vi "Perform Action.vi"(8 "error in (no error)":errorcluster, 10 "Input":variant, 11 "DIO DAQmx Fixed Freq PWM CFG in":refnum<class "CO DAQmx Fixed Freq PWM CFG.lvclass">) -> (0 "error out":errorcluster, 2 "Output":variant, 3 "DIO DAQmx Fixed Freq PWM CFG out":refnum<class "CO DAQmx Fixed Freq PWM CFG.lvclass">)   [LabVIEW 2023, in "CO DAQmx Fixed Freq PWM CFG.lvclass"]
uses:
  CO DAQmx Fixed Freq PWM CFG.lvclass
  <resource>/objmgr/daqmx.rc
  DAQmx/DAQmx Base CFG/DAQmx Base CFG.lvclass
  Configuration/Configuration Semaphore/CFG Semaphore.lvclass
  <vilib>/Utility/error.llb/Error Cluster From Error Code.vi
  <vilib>/ErrorRing/Error Ring.xnode
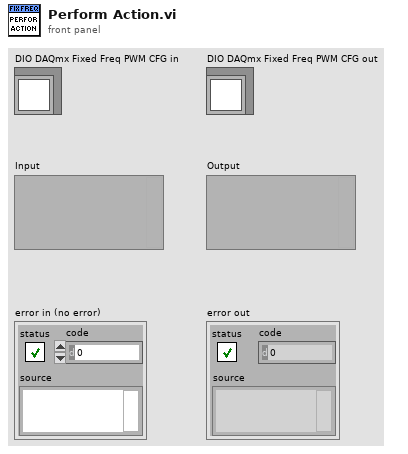
[diagram p1: front panel]
types:
  T1 = typedef "Semaphore RefNum" = refnum<k1>
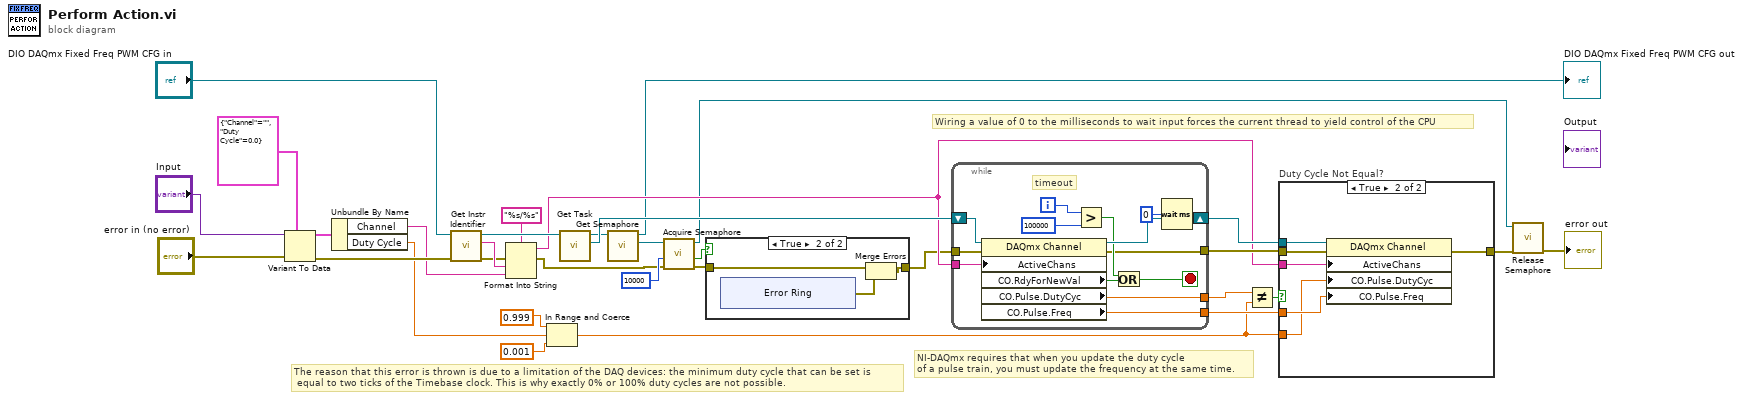
[diagram p0: block diagram]
diagram:
  # "The reason that this error is thrown is due to a limitation of the DAQ devices: the minimum duty cycle that can be set is\n equal to two ticks of the Timebase clock. This is why exactly 0% or 100% duty cycles are not possible."
  # "Wiring a value of 0 to the milliseconds to wait input forces the current thread to yield control of the CPU"
  # "NI-DAQmx requires that when you update the duty cycle\nof a pulse train, you must update the frequency at the same time."
  n1 = Variant To Data(error in="error in (no error)", type=cluster{"Channel":string, "Duty Cycle":dbl} {"Channel"="", "Duty Cycle"=0.0}, Variant="Input") -> (data=w31:cluster{"Channel":string, "Duty Cycle":dbl}, error out=w32:errorcluster)
  n2 = Unbundle By Name(w31) -> ("Channel"=w27:string, "Duty Cycle"=w19:dbl)
  n3 = call-dynamic "Get Instr Identifier.vi"("error in"=w32, "Configuration Base in"="DIO DAQmx Fixed Freq PWM CFG in") -> ("error out"=w26:errorcluster, "Instr Ident"=w28:string, "Configuration Base out"=w30:refnum<class "CO DAQmx Fixed Freq PWM CFG.lvclass">)  [unwired: 7 in]
  n4 = Format Into String(format string="%s/%s", error in=w26, w28, w27) -> (resulting string=w21:string, error out=w1:errorcluster)  [unwired: 1 in]
  n5 = In Range and Coerce(upper limit=0.999, x=w19, lower limit=0.001) -> (coerced(x)=w4:dbl)  [unwired: 1 out]
  n6 = call "Get Task.vi"("DAQmx Base CFG in"=w30) -> ("Task"=w23:refnum<k21>, "DAQmx Base CFG out"=w14:refnum<class "CO DAQmx Fixed Freq PWM CFG.lvclass">)  [unwired: 9 in]
  n7 = call "Get Semaphore.vi"("CFG Base in"=w14) -> ("Semaphore"=w13:T1, "CFG Base out"=→"DIO DAQmx Fixed Freq PWM CFG out":refnum<class "CO DAQmx Fixed Freq PWM CFG.lvclass">)  [unwired: 9 in]
  n8 = call <vilib>:"Acquire Semaphore.vi"("error in (no error)"=w1, "ms timeout (-1)"=10000, "semaphore"=w13) -> ("error out"=w7:errorcluster, "timed out"=w6:bool, "semaphore out"=w10:T1)  [unwired: 2 in]
  n9 = case shown="True" w6 {
    tunnel: w7 -> [w34 w36]
    tunnel: [w34 w35] -> w5
    frame False {
    }
    frame True {
      n10 = xnode "Error Ring"() -> ("error out"=w37:errorcluster)
      n11 = Merge Errors(w36, w37) -> (w35:errorcluster)
    }
  }
  n12 = while {
    tunnel: [w54] -> w18
    tunnel: w5 -> [w53]
    tunnel: [w51] -> w20
    tunnel: w21 -> [w50]
    shift-right: [w55] -> w25
    shift-left: w23 -> [w52]
    tunnel: [w43] -> w22
    i -> [w48]
    stop <- w46 stop-if-true
    # "timeout"
    n13 = property class="DAQmx Channel"(reference=w52, error in=w53, "ActiveChans"=w50) -> (reference out=w55:refnum<k21>, error out=w43:errorcluster, "CO.RdyForNewVal"=w49:bool, "CO.Pulse.DutyCyc"=w54:dbl, "CO.Pulse.Freq"=w51:dbl)
    n14 = Greater?(x=w48, y=100000) -> (0:w45:bool)
    n15 = Or(x=w45, y=w49) -> (x .or. y?=w46:bool)
    n16 = Wait (ms)(milliseconds to wait=u32 0) -> ()  [unwired: 1 out]
  }
  n17 = Not Equal?(x=w18, y=w4) -> (x != y?=w24:bool)
  n18 = case "Duty Cycle Not Equal?" shown="True" w24 {
    tunnel: [w56 w62] -> w12
    tunnel: w22 -> [w56 w61]
    tunnel: w25 -> [_ w60]
    tunnel: w21 -> [_ w59]
    tunnel: w20 -> [_ w58]
    tunnel: w4 -> [_ w57]
    frame False {
    }
    frame True {
      n19 = property class="DAQmx Channel"(reference=w60, error in=w61, "ActiveChans"=w59, "CO.Pulse.DutyCyc"=w57, "CO.Pulse.Freq"=w58) -> (error out=w62:errorcluster)  [unwired: 1 out]
    }
  }
  n20 = call <vilib>:"Release Semaphore.vi"("error in (no error)"=w12, "semaphore"=w10) -> ("error out"=→"error out":errorcluster)  [unwired: 4 in, 1 out]
